vi "Convert HW number to Data Bytes.vi"(11 "HW part number":string) -> (3 "ASCII":u8[](array[numeric]) format="%.0x")   [LabVIEW 2023]
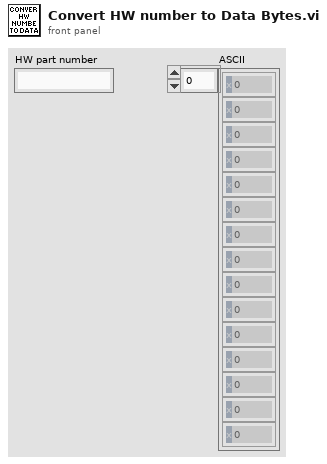
[diagram p1: front panel]
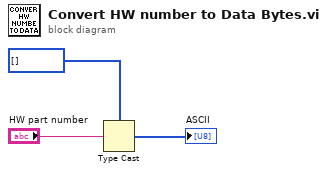
[diagram p0: block diagram]
diagram:
  n1 = Type Cast(type=u8[] [] ("DATA[5]"), x="HW part number") -> (*(type *) &x=→"ASCII":u8[])
